vi "Vision Acquisition Image Logging.vi"(4 "File Settings":T2, 6 "Close":bool, 7 "Log Image":bool, 8 "error in (no error)":errorcluster, 10 "Image Logging Path":path, 11 "Image In":T1) -> (0 "error out":errorcluster, 3 "Image Logging Path Out":path)   [LabVIEW 2019, in "GaitDAQ UI.lvlib"]
uses:
  GaitDAQ UI.lvlib
  <vilib>/vision/Image Controls.llb/IMAQ Image.ctl
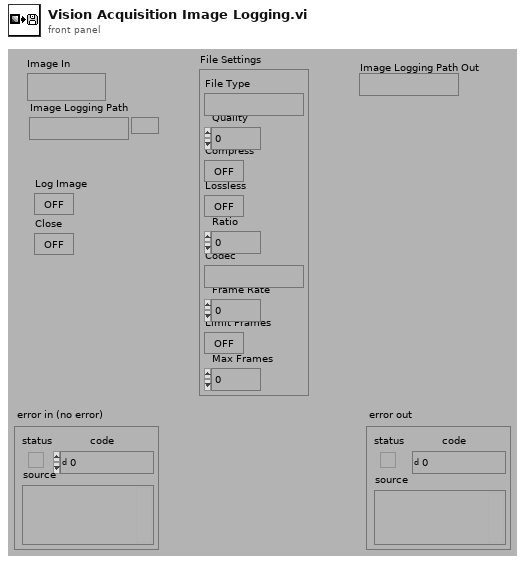
[diagram p1: front panel]
types:
  T1 = typedef "IMAQ Image.ctl" = refnum<image>
  T2 = cluster{"File Type":string, "Quality":u32, "Compress":bool, "Lossless":bool, "Ratio":sgl, "Codec":string, "Frame Rate":u32, "Limit Frames":bool, "Max Frames":u32}
  T3 = typedef "Image Type" = u32
  T4 = typedef "IMAQ AVI2 Refnum.ctl" = refnum<k20>
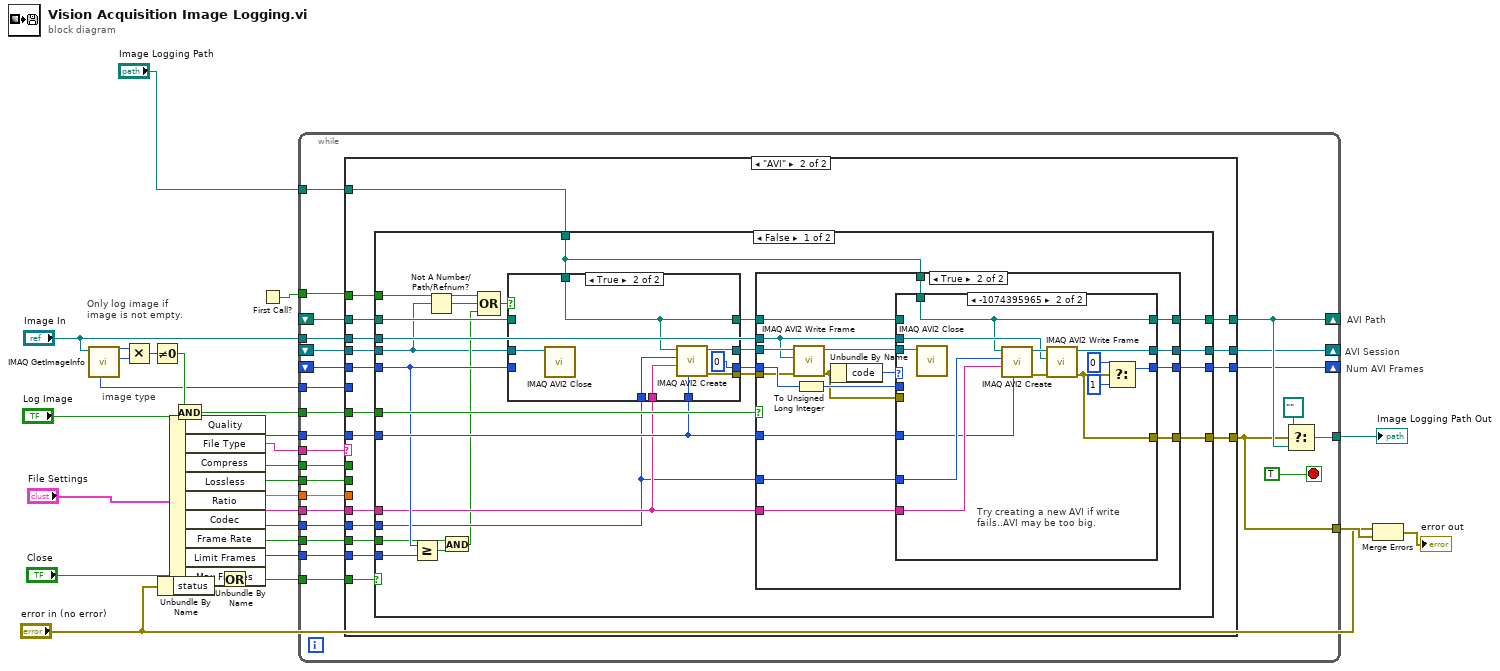
[diagram p0: block diagram]
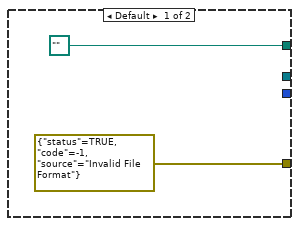
[diagram p2: hidden frame]
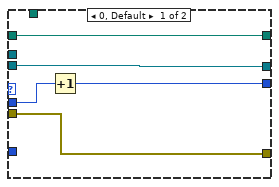
[diagram p4: hidden frame]
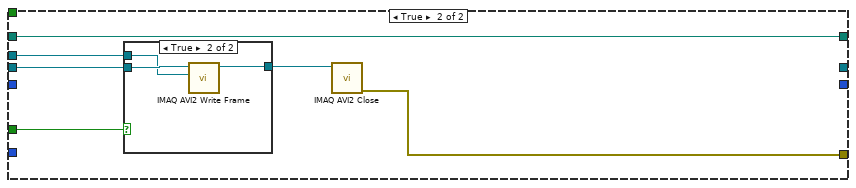
[diagram p6: hidden frame]
diagram:
  # "image type"
  # "Only log image if image is not empty."
  # "Num AVI Frames"
  # "AVI Session"
  # "AVI Path"
  n1 = call "IMAQ GetImageInfo"("Image"="Image In") -> ("Y Resolution"=w14:i32, "X Resolution"=w15:i32, "Image Type"=w8:T3)  [unwired: 1 in, 7 out]
  n2 = Multiply(x=w15, y=w14) -> (x*y=w16:i32)
  n3 = Not Equal To 0?(x=w16) -> (x != 0?=w17:bool)
  n4 = Unbundle By Name("error in (no error)") -> ("status"=w6:bool)
  n5 = Unbundle By Name("File Settings") -> ("Quality"=w20:u32, "File Type"=w3:string, "Compress"=w21:bool, "Lossless"=w22:bool, "Ratio"=w23:sgl, "Codec"=w24:string, "Frame Rate"=w25:u32, "Limit Frames"=w26:bool, "Max Frames"=w27:u32)
  n6 = And(x=w17, y="Log Image") -> (x .and. y?=w18:bool)
  n7 = Or(x="Close", y=w6) -> (x .or. y?=w5:bool)
  n8 = First Call?() -> (First Call?: T/F=w2:bool)
  n9 = while {
    tunnel: "Image In" -> [w51]
    tunnel: w3 -> [w50]
    shift-right: [w49] -> _
    shift-left: _ -> [w44]
    tunnel: w18 -> [w47]
    shift-right: [w46] -> _
    shift-left: _ -> [w45]
    shift-right: [w42] -> _
    shift-left: _ -> [w43]
    tunnel: [w41] -> w11
    tunnel: w20 -> [w40]
    tunnel: w21 -> [w39]
    tunnel: w22 -> [w38]
    tunnel: w23 -> [w37]
    tunnel: w24 -> [w36]
    tunnel: w25 -> [w35]
    tunnel: w26 -> [w34]
    tunnel: w27 -> [w33]
    tunnel: [w32] -> w10
    tunnel: w5 -> [w31]
    tunnel: w8 -> [w30]
    tunnel: "Image Logging Path" -> [w29]
    tunnel: w2 -> [w28]
    stop <- TRUE stop-if-true
    n10 = case shown="\"AVI\"" w50 {
      tunnel: w51 -> [_ w69]
      tunnel: [path "" w63] -> w49
      tunnel: [errorcluster {"status"=TRUE, "code"=-1, "source"="Invalid File Format"} ("error out") w67] -> w32
      tunnel: w40 -> [_ w62]
      tunnel: w28 -> [_ w64]
      tunnel: w47 -> [_ w66]
      tunnel: [_ w68] -> w46
      tunnel: w45 -> [_ w71]
      tunnel: w44 -> [_ w70]
      tunnel: w43 -> [_ w61]
      tunnel: [_ w65] -> w42
      tunnel: w39 -> [_ _]
      tunnel: w38 -> [_ _]
      tunnel: w37 -> [_ _]
      tunnel: w36 -> [_ w60]
      tunnel: w35 -> [_ w59]
      tunnel: w34 -> [_ w58]
      tunnel: w33 -> [_ w57]
      tunnel: w31 -> [_ w56]
      tunnel: w30 -> [_ _]
      tunnel: w29 -> [_ w55]
      frame Default {
      }
      frame "AVI" {
        n11 = case shown="False" w56 {
          tunnel: w71 -> [w74 w151]
          tunnel: w70 -> [w95 w148]
          tunnel: w69 -> [w93 w150]
          tunnel: [w91 _] -> w68
          tunnel: [w90 w146] -> w67
          tunnel: w66 -> [w89 w149]
          tunnel: [w88 _] -> w65
          tunnel: w64 -> [w87 _]
          tunnel: [w83 w148] -> w63
          tunnel: w62 -> [w82 _]
          tunnel: w61 -> [w81 _]
          tunnel: w60 -> [w79 _]
          tunnel: w59 -> [w78 _]
          tunnel: w58 -> [w77 _]
          tunnel: w57 -> [w76 _]
          tunnel: w55 -> [w72 _]
          frame False {
            n12 = Greater Or Equal?(x=w81, y=w76) -> (x >= y?=w85:bool)
            n13 = Not A Number/Path/Refnum?(number/path/refnum=w74) -> (NaN/Path/Refnum?=w73:bool)
            n14 = And(x=w77, y=w85) -> (x .and. y?=w75:bool)
            n15 = Compound Arithmetic op=OR(w87, w73, w75) -> (w86:bool)
            n16 = case shown="True" w86 {
              tunnel: [w136 w138] -> w84
              tunnel: [w137 w141] -> w94
              tunnel: [_ w142] -> w92
              tunnel: w74 -> [w137 w144]
              tunnel: w95 -> [w136 _]
              tunnel: w78 -> [_ w140]
              tunnel: w79 -> [_ w139]
              tunnel: w82 -> [_ w143]
              tunnel: w81 -> [w135 _]
              tunnel: [w135 u32 0 ("f")] -> w80
              tunnel: w72 -> [_ w138]
              frame False {
              }
              frame True {
                n17 = call "IMAQ AVI2 Close"("AVI Refnum"=w144) -> ()  [unwired: 1 in, 10 out]
                n18 = call "IMAQ AVI2 Create"("Quality"=w143, "Codec"=w139, "Frames Per Second"=w140, "AVI Path"=w138) -> ("error out"=w142:errorcluster, "AVI Refnum"=w141:T4)  [unwired: 1 in, 5 out]
              }
            }
            n19 = case shown="True" w89 {
              tunnel: w94 -> [w98 w105]
              tunnel: w93 -> [_ w104]
              tunnel: w92 -> [w97 w106]
              tunnel: [w98 w113] -> w91
              tunnel: [w97 w112] -> w90
              tunnel: w80 -> [w99 w116]
              tunnel: [w99 w114] -> w88
              tunnel: w78 -> [_ w111]
              tunnel: w84 -> [w96 w110]
              tunnel: [w96 w109] -> w83
              tunnel: w79 -> [_ w108]
              tunnel: w82 -> [_ w107]
              tunnel: w72 -> [_ w100]
              frame False {
              }
              frame True {
                n20 = call "IMAQ AVI2 Write Frame"("error in (no error)"=w106, "Image"=w104, "AVI Refnum"=w105) -> ("error out"=w101:errorcluster, "AVI Refnum (duplicate)"=w103:T4)  [unwired: 7 out]
                n21 = To Unsigned Long Integer(number=w116) -> (unsigned 32bit integer=w115:u32)
                n22 = Unbundle By Name(w101) -> ("code"=w102:i32)
                n23 = case shown="-1074395965" w102 {
                  tunnel: w103 -> [w119 w131]
                  tunnel: w115 -> [w121 _]
                  tunnel: [w120 w133] -> w114
                  tunnel: [w119 w123] -> w113
                  tunnel: [w117 w124] -> w112
                  tunnel: w111 -> [_ w130]
                  tunnel: w110 -> [w118 _]
                  tunnel: [w118 w122] -> w109
                  tunnel: w108 -> [_ w129]
                  tunnel: w107 -> [_ w128]
                  tunnel: w104 -> [_ w126]
                  tunnel: w101 -> [w117 _]
                  tunnel: w100 -> [_ w122]
                  frame 0, Default {
                    n24 = Increment(x=w121) -> (x+1=w120:u32)
                  }
                  frame -1074395965 {
                    # "Try creating a new AVI if write fails..AVI may be too big."
                    n25 = call "IMAQ AVI2 Close"("AVI Refnum"=w131) -> ()  [unwired: 1 in, 10 out]
                    n26 = call "IMAQ AVI2 Create"("Quality"=w128, "Codec"=w129, "Frames Per Second"=w130, "AVI Path"=w122) -> ("error out"=w125:errorcluster, "AVI Refnum"=w127:T4)  [unwired: 1 in, 5 out]
                    n27 = call "IMAQ AVI2 Write Frame"("error in (no error)"=w125, "Image"=w126, "AVI Refnum"=w127) -> ("error out"=w124:errorcluster, "AVI Refnum (duplicate)"=w123:T4)  [unwired: 7 out]
                    n28 = Select(t=u32 0, s=w124, f=u32 1) -> (s? t:f=w133:u32)
                  }
                }
              }
            }
          }
          frame True {
            n29 = case shown="True" w149 {
              tunnel: w151 -> [w152 w155]
              tunnel: w150 -> [_ w154]
              tunnel: [w152 w153] -> w147
              frame False {
              }
              frame True {
                n30 = call "IMAQ AVI2 Write Frame"("Image"=w154, "AVI Refnum"=w155) -> ("AVI Refnum (duplicate)"=w153:T4)  [unwired: 1 in, 8 out]
              }
            }
            n31 = call "IMAQ AVI2 Close"("AVI Refnum"=w147) -> ("error out"=w146:errorcluster)  [unwired: 1 in, 9 out]
          }
        }
      }
    }
    n32 = Select(t=path "", s=w32, f=w49) -> (s? t:f=w41:path)
  }
  "Image Logging Path Out" <- w11
  n33 = Merge Errors("error in (no error)", w10) -> (→"error out":errorcluster)
